vi "数据查询_报警信息.vi"() -> ()   [LabVIEW 2016]
uses:
  <vilib>/Utility/sysdir.llb/System Directory Type.ctl
  <vilib>/Utility/miscctls.llb/LVPointTypeDef.ctl
  <vilib>/addons/database/Connection.llb/DB Tools Open Connec (String).vi
  <vilib>/addons/database/_DB Variant To Data/Database Variant To Data.xnode
  <vilib>/addons/database/NI_Database_API.lvlib
panel:
  in  "搜索按钮":bool
  in  "布尔":bool
  in  "下拉列表":u16(ring) items=["全部", "氨氮", "总磷总氮", "多参数", "CodMn", "其他"]
  out "error out":errorcluster caption="错误输出"
  in  "error in (no error)":errorcluster caption="错误输入（无错误）"
  out "数据表":string[][](table)
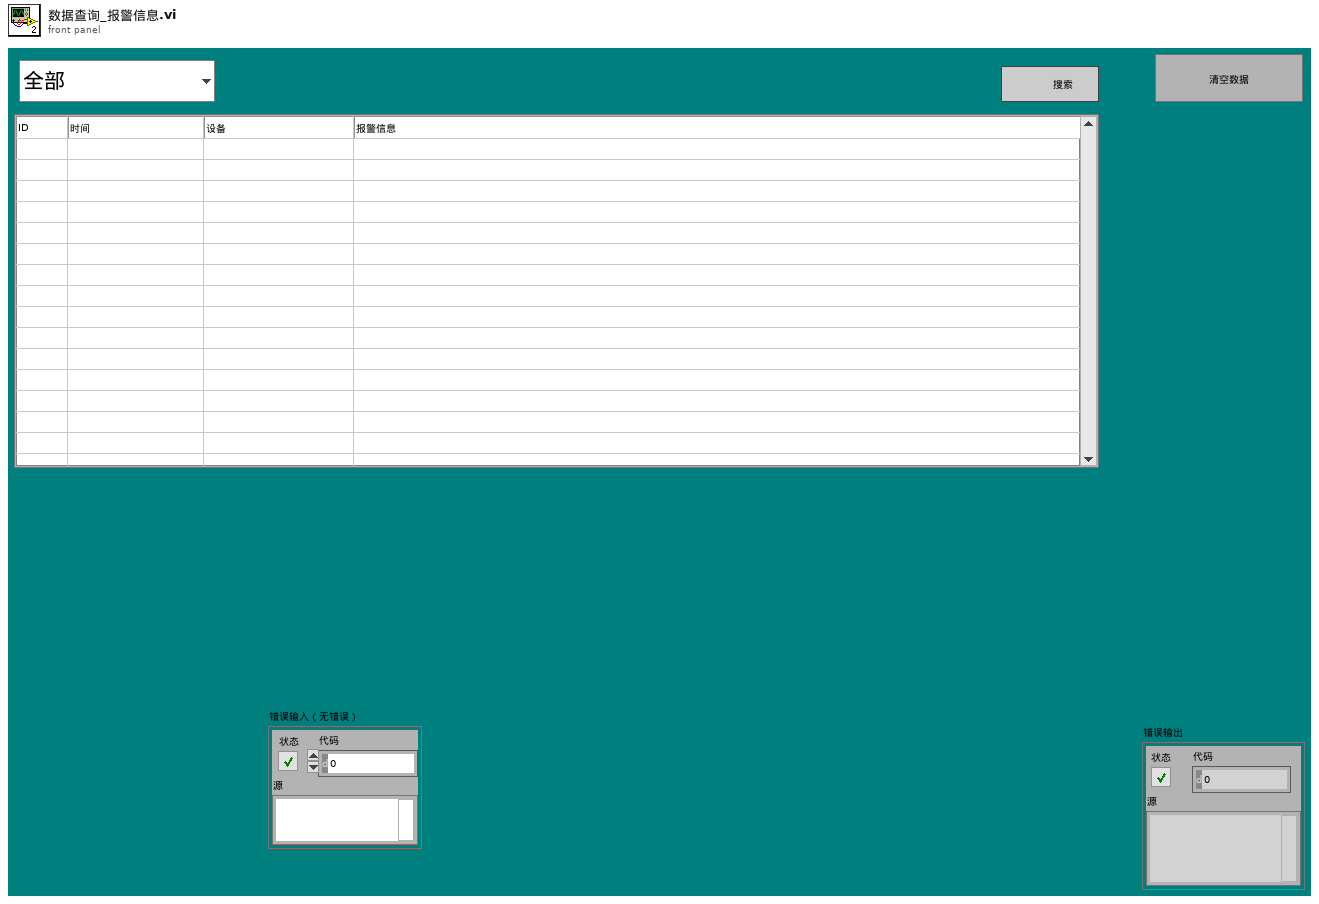
[diagram p1: front panel]
types:
  T1 = typedef "System Directory Type.ctl" = i32
  T2 = typedef "LVPointTypeDef.ctl" = cluster{"Horizontal":i16, "Vertical":i16}
  T3 = typedef "NI_Database_API.lvlib/Conn ObjectReference.ctl" = refnum<k1>
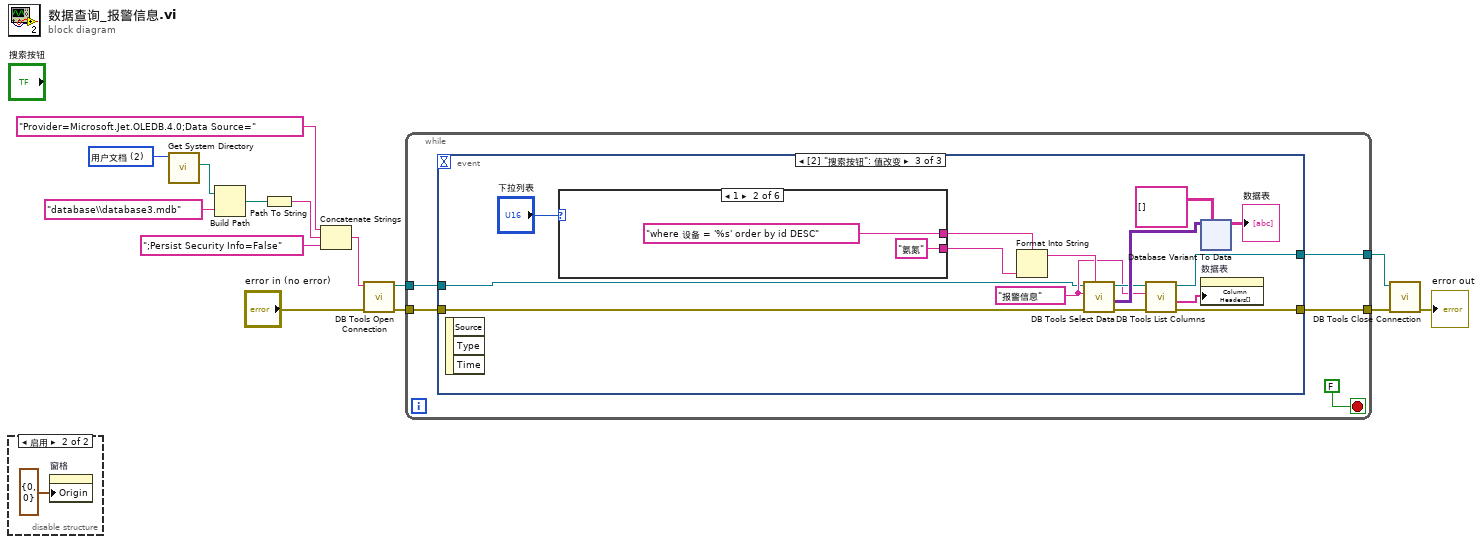
[diagram p0: block diagram]
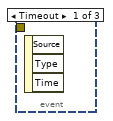
[diagram p3: hidden frame]
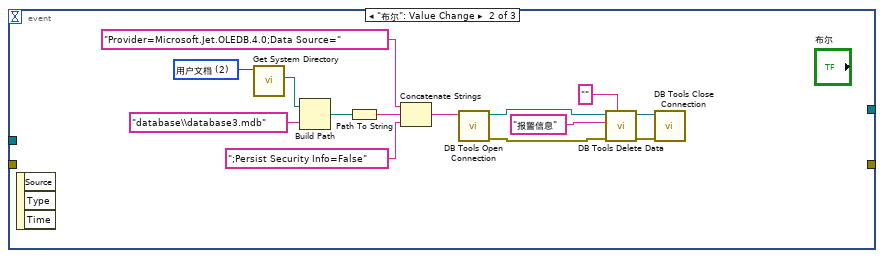
[diagram p4: hidden frame]
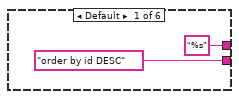
[diagram p5: hidden frame]
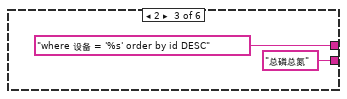
[diagram p6: hidden frame]
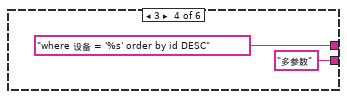
[diagram p7: hidden frame]
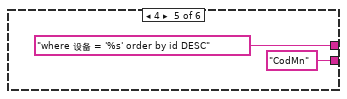
[diagram p8: hidden frame]
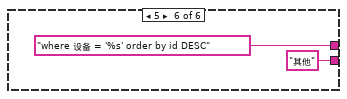
[diagram p9: hidden frame]
diagram:
  w10 = T1 2 items=["用户目录"=0, "用户桌面"=1, "用户文档"=2, "用户应用程序数据"=3, "用户设置"=4, "用户临时目录"=5, "公共文档"=6, "公共应用程序数据"=7, "公共设置"=8, "公共缓存"=13, "系统核心库"=9, "系统安装库"=10, "应用程序文件"=11, "启动盘根目录"=12] ("system directory type")
  n1 = disable-structure shown="启用" {
    frame Disabled {
    }
    frame Enabled {
      n2 = property on="窗格" class="Pane"("Origin"=T2 {"Horizontal"=0, "Vertical"=0} ("原点")) -> ()  [unwired: 2 in, 2 out]
    }
  }
  n3 = call <vilib>:"Get System Directory.vi"("system directory type"=w10) -> ("system directory"=w9:path)  [unwired: 10 in]
  n4 = Build Path(base path=w9, name or relative path="database\\database3.mdb" ("名称或相对路径")) -> (appended path=w11:path)
  n5 = Path To String(path=w11) -> (string=w12:string)
  n6 = Concatenate Strings("Provider=Microsoft.Jet.OLEDB.4.0;Data Source=", w12, ";Persist Security Info=False") -> (w14:string)
  n7 = call-poly <vilib>:"DB Tools Open Connection.vi"("error in (no error)"="error in (no error)", "connection information"=w14) -> ("error out"=w4:errorcluster, "connection reference"=w5:T3)  [unwired: 6 in]
  n8 = while {
    tunnel: w5 -> [w19]
    tunnel: w4 -> [w18]
    tunnel: [w17] -> w2
    tunnel: [w16] -> w1
    stop <- FALSE stop-if-true
    n9 = event shown="[2] \"搜索按钮\": 值改变" {
      selector: _ -> [_ _ _]
      dyn-events: _ -> [_ _ _]
      timeout: _ -> [_ _ _]
      tunnel: w19 -> [_ _ w38]
      tunnel: w18 -> [_ _ w37]
      tunnel: [_ _ w36] -> w17
      tunnel: [_ _ w35] -> w16
      event Timeout {
        n10 = event-data() -> ()  [unwired: 1 in, 3 out]
      }
      event "布尔": Value Change {
        w25 = T1 2 items=["用户目录"=0, "用户桌面"=1, "用户文档"=2, "用户应用程序数据"=3, "用户设置"=4, "用户临时目录"=5, "公共文档"=6, "公共应用程序数据"=7, "公共设置"=8, "公共缓存"=13, "系统核心库"=9, "系统安装库"=10, "应用程序文件"=11, "启动盘根目录"=12] ("system directory type")
        n11 = event-data() -> ()  [unwired: 1 in, 3 out]
        n12 = call <vilib>:"Get System Directory.vi"("system directory type"=w25) -> ("system directory"=w26:path)  [unwired: 10 in]
        n13 = Build Path(base path=w26, name or relative path="database\\database3.mdb" ("名称或相对路径")) -> (appended path=w24:path)
        n14 = Path To String(path=w24) -> (string=w23:string)
        n15 = Concatenate Strings("Provider=Microsoft.Jet.OLEDB.4.0;Data Source=", w23, ";Persist Security Info=False") -> (w28:string)
        n16 = call-poly <vilib>:"DB Tools Open Connection.vi"("connection information"=w28) -> ("error out"=w30:errorcluster, "connection reference"=w29:T3)  [unwired: 7 in]
        n17 = call <vilib>:"DB Tools Delete Data.vi"("condition"="", "error in (no error)"=w30, "table"="报警信息", "connection reference"=w29) -> ("error out"=w32:errorcluster, "connection reference out"=w31:T3)  [unwired: 6 in]
        n18 = call <vilib>:"DB Tools Close Connection.vi"("error in (no error)"=w32, "connection reference"=w31) -> ()  [unwired: 5 in, 1 out]
      }
      event "搜索按钮": Value Change {
        w39 = "报警信息" ("组合框")
        n19 = event-data() -> ()  [unwired: 1 in, 3 out]
        n20 = case shown="1" "下拉列表" {
          tunnel: ["%s" ("格式字符串") "where 设备 = '%s' order by id DESC" ("格式字符串") "where 设备 = '%s' order by id DESC" ("格式字符串") "where 设备 = '%s' order by id DESC" ("格式字符串") "where 设备 = '%s' order by id DESC" ("格式字符串") "where 设备 = '%s' order by id DESC" ("格式字符串")] -> w47
          tunnel: ["order by id DESC" ("格式字符串") "氨氮" ("格式字符串") "总磷总氮" ("格式字符串") "多参数" ("格式字符串") "CodMn" ("格式字符串") "其他" ("格式字符串")] -> w48
          frame Default {
          }
          frame 1 {
          }
          frame 2 {
          }
          frame 3 {
          }
          frame 4 {
          }
          frame 5 {
          }
        }
        n21 = Format Into String(format string=w47, w48) -> (resulting string=w49:string)  [unwired: 2 in, 1 out]
        n22 = call <vilib>:"DB Tools Select Data.vi"("condition"=w49, "error in (no error)"=w37, "table"=w39, "connection reference"=w38) -> ("error out"=w42:errorcluster, "data"=w45:variant[][], "connection reference out"=w43:T3)  [unwired: 2 in]
        n23 = call <vilib>:"DB Tools List Columns.vi"("error in (no error)"=w42, "table"=w39, "connection reference"=w43) -> ("error out"=w35:errorcluster, "columns"=w40:string[], "connection reference out"=w36:T3)  [unwired: 1 in, 1 out]
        n24 = xnode "Database Variant To Data"("database variant"=w45, "type"=string[][] []) -> ("data"=→"数据表":string[][])  [unwired: 1 in, 1 out]
        n25 = property on="数据表" class="Tbl (严格)"("Column Headers[]"=w40) -> ()  [unwired: 2 in, 2 out]
      }
    }
  }
  n26 = call <vilib>:"DB Tools Close Connection.vi"("error in (no error)"=w1, "connection reference"=w2) -> ("error out"=→"error out":errorcluster)  [unwired: 5 in]
